vi "subCloseCurrentProject.vi"(8 "error in (no error)":errorcluster, 11 "BuildManager in":refnum<class "BuildManager.lvclass">) -> (0 "error out":errorcluster, 3 "BuildManager out":refnum<class "BuildManager.lvclass">)   [LabVIEW 2019, in "SolutionBuilder.lvlib" / "BuildManager.lvclass"]
uses:
  BuildManager.lvclass
  BuildManager.lvclass/BuildManager.ctl
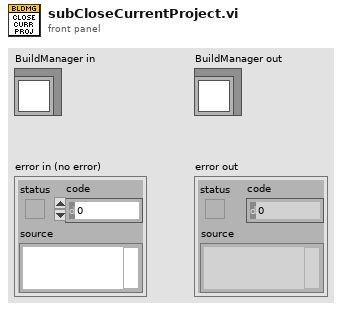
[diagram p1: front panel]
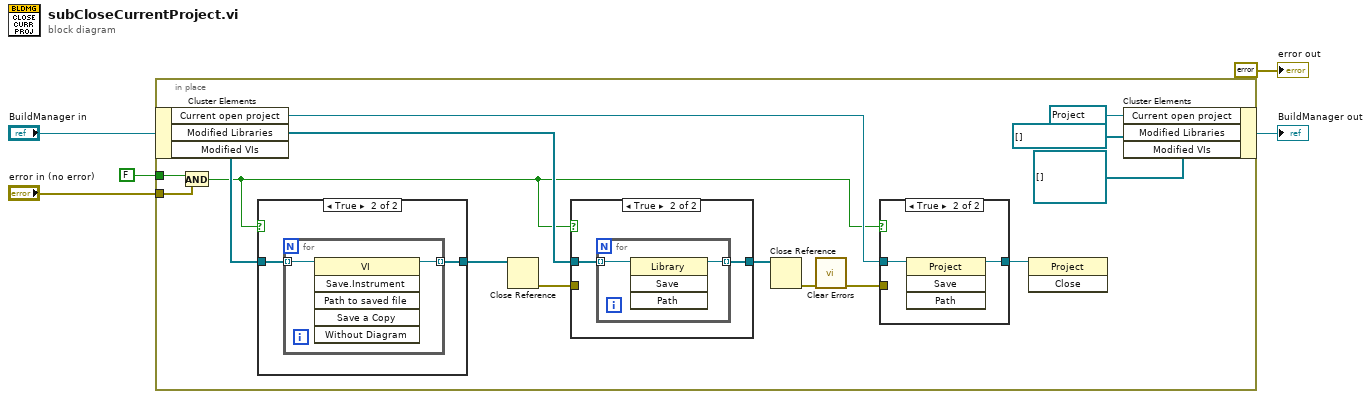
[diagram p0: block diagram]
diagram:
  n1 = in-place {
    in-place-border: "error in (no error)" -> [w8]
    in-place-border: FALSE -> [w7]
    n2 = in-place-cluster #1("BuildManager in") -> ("Current open project"=w11:refnum<vi>, "Modified Libraries"=w14:refnum<vi>[], "Modified VIs"=w16:refnum<vi>[])
    n3 = And(x=w7, y=w8) -> (x .and. y?=w6:bool)
    n4 = case shown="True" w6 {
      tunnel: w16 -> [w29 w31]
      tunnel: [w29 w30] -> w15
      frame False {
      }
      frame True {
        n5 = for {
          tunnel: w31 -> [w33] mode=indexing
          tunnel: [w32] -> w30 mode=indexing
          n6 = invoke class="VI" method="Save.Instrument"(reference=w33) -> (reference out=w32:refnum<vi>)  [unwired: 5 in, 5 out]
        }
      }
    }
    n7 = Close Reference(reference=w15) -> (error out=w13:errorcluster)  [unwired: 1 in]
    n8 = case shown="True" w6 {
      tunnel: w14 -> [w24 w26]
      tunnel: [w24 w25] -> w12
      tunnel: w13 -> [_ _]
      frame False {
      }
      frame True {
        n9 = for {
          tunnel: w26 -> [w28] mode=indexing
          tunnel: [w27] -> w25 mode=indexing
          n10 = invoke class="Library" method="Save"(reference=w28) -> (reference out=w27:refnum<vi>)  [unwired: 3 in, 3 out]
        }
      }
    }
    n11 = Close Reference(reference=w12) -> (error out=w17:errorcluster)  [unwired: 1 in]
    n12 = call <vilib>:"Clear Errors.vi"("error in (no error)"=w17) -> ("error out"=w10:errorcluster)  [unwired: 5 in, 1 out]
    n13 = case shown="True" w6 {
      tunnel: w11 -> [w21 w23]
      tunnel: [w21 w22] -> w9
      tunnel: w10 -> [_ _]
      frame False {
      }
      frame True {
        n14 = invoke class="Project" method="Save"(reference=w23) -> (reference out=w22:refnum<vi>)  [unwired: 3 in, 3 out]
      }
    }
    n15 = invoke class="Project" method="Close"(reference=w9) -> ()  [unwired: 2 in, 3 out]
    n16 = in-place-cluster #1("Current open project"=refnum<vi> refnum, "Modified Libraries"=refnum<vi>[] [], "Modified VIs"=refnum<vi>[] []) -> (→"BuildManager out":refnum<class "BuildManager.lvclass">)
  }
  "error out" <- errorcluster {"status"=FALSE, "code"=0, "source"=""} ("error out")
